vi "check for tags.vi"(1 "Info":T1={"Make"="Canon\u0000", "Model"="Canon PowerShot A495\u0000", "Orientation"=0, "Date"=timestamp(0 s since 1904-01-01), "Width"=0, "Height"=0, "Square?"=FALSE, "File Name"="Canon\u0000", "Extension"="Canon\u0000", "Valid?"=FALSE, "Path"=path "", "size"=0, "No Ext?"=FALSE, "prefix?"=FALSE, "Tag"="", "Name Type"=enum."Event Sufix", "Projection Type"="Canon\u0000"}) -> (0 "Info out":T1={"Make"="Canon\u0000", "Model"="Canon PowerShot A495\u0000", "Orientation"=0, "Date"=timestamp(0 s since 1904-01-01), "Width"=0, "Height"=0, "Square?"=FALSE, "File Name"="Canon\u0000", "Extension"="Canon\u0000", "Valid?"=FALSE, "Path"=path "", "size"=0, "No Ext?"=FALSE, "prefix?"=FALSE, "Tag"="", "Name Type"=enum."Event Sufix", "Projection Type"="Canon\u0000"})   [LabVIEW 2023, in "File Classes.lvlib" / "Picture File.lvclass"]
uses:
  Picture File.lvclass
  Controls/exif data cluster.ctl
  Controls/rename type enum.ctl
  File Classes.lvlib
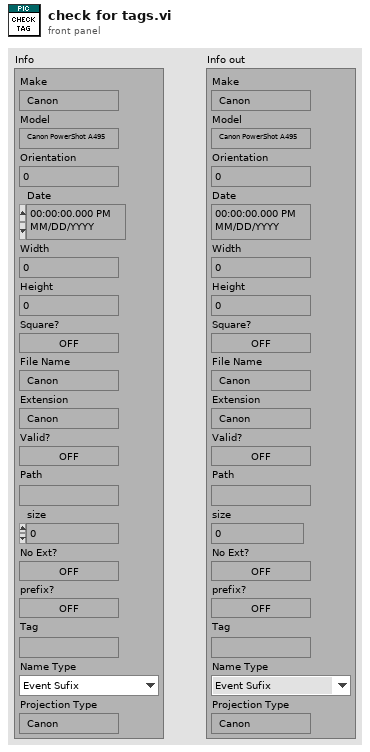
[diagram p1: front panel]
types:
  T1 = typedef "File Classes.lvlib/exif data cluster.ctl" = cluster{"Make":string, "Model":string, "Orientation":u16, "Date":timestamp, "Width":u16, "Height":u16, "Square?":bool, "File Name":string, "Extension":string, "Valid?":bool, "Path":path, "size":i64, "No Ext?":bool, "prefix?":bool, "Tag":string, "Name Type":T2, "Projection Type":string}
  T2 = typedef "File Classes.lvlib/rename type enum.ctl" = enum16{"Date & Time (Default)", "Model Sufix", "Event Sufix", "Model & Event Sufix"}
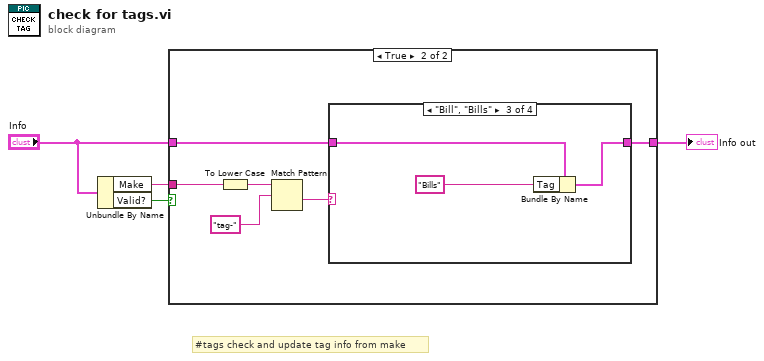
[diagram p0: block diagram]
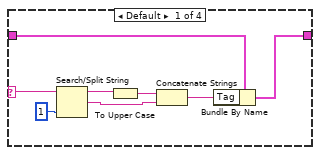
[diagram p3: hidden frame]
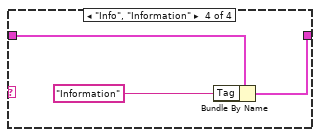
[diagram p5: hidden frame]
diagram:
  # "#tags check and update tag info from make"
  n1 = Unbundle By Name("Info") -> ("Make"=w4:string, "Valid?"=w1:bool)
  n2 = case shown="True" w1 {
    tunnel: w4 -> [_ w11]
    tunnel: "Info" -> [w5 w7]
    tunnel: [w5 w6] -> w2
    frame False {
    }
    frame True {
      n3 = To Lower Case(string=w11) -> (all lower case string=w10:string)
      n4 = Match Pattern(string=w10, regular expression="tag-") -> (after substring=w8:string)  [unwired: 1 in, 3 out]
      n5 = case shown="\"Bill\", \"Bills\"" w8 {
        selector: w8 -> [w17 _ _ _]
        tunnel: [w18 w20 w22 w25] -> w6
        tunnel: w7 -> [w19 w20 w23 w26]
        frame Default {
          n6 = Search/Split String(string=w17, offset (0)=1) -> (substring before match=w15:string, match + rest of string=w13:string)  [unwired: 1 in, 1 out]
          n7 = To Upper Case(1:w15) -> (0:w14:string)
          n8 = Concatenate Strings(w14, w13) -> (w12:string)
          n9 = Bundle By Name(cluster=w19, "Tag"=w12) -> (w18:T1)
        }
        frame "" {
        }
        frame "Bill", "Bills" {
          n10 = Bundle By Name(cluster=w23, "Tag"="Bills") -> (w22:T1)
        }
        frame "Info", "Information" {
          n11 = Bundle By Name(cluster=w26, "Tag"="Information") -> (w25:T1)
        }
      }
    }
  }
  "Info out" <- w2
